vi "Command.vi"(7 "Cryo Idx":i32, 8 "error in (no error)":errorcluster, 9 "Options":string, 10 "Command":T1 items=["STATUS", "COOLER", "E", "ERROR", "KD", "KI", "KP", "LOGIN", "LOGOUT", "MODE", "P", "PWOUT", "SENSOR", "TC", "TEMP RJ", "TTARGET", "VERSION"], 11 "CryoCoolerAVC in":refnum<class "CryoCoolerAVC.lvclass">) -> (0 "error out":errorcluster, 2 "Response":string[](array[string]), 3 "CryoCoolerAVC out":refnum<class "CryoCoolerAVC.lvclass">)   [LabVIEW 2024, in "CryoCoolerAVC.lvclass"]
uses:
  CryoCoolerAVC.lvclass
  CryoCoolerAVC Command enum.ctl
  CryoCoolerAVC.lvclass/CryoCoolerAVC.ctl
  Cryo Cooler.lvclass
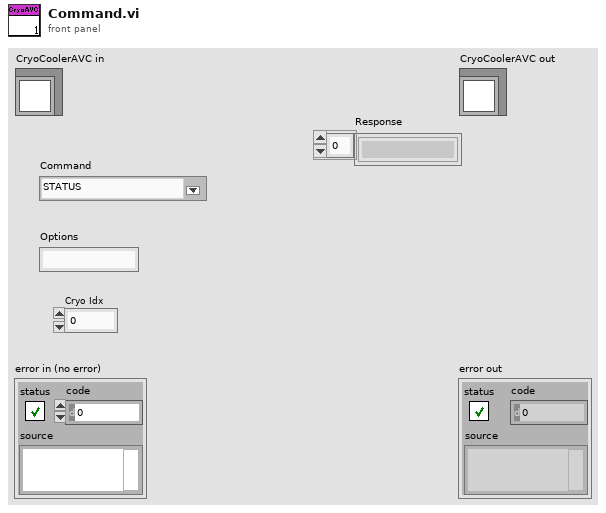
[diagram p1: front panel]
types:
  T1 = typedef "CryoCoolerAVC.lvclass/CryoCoolerAVC Command enum.ctl" = u16
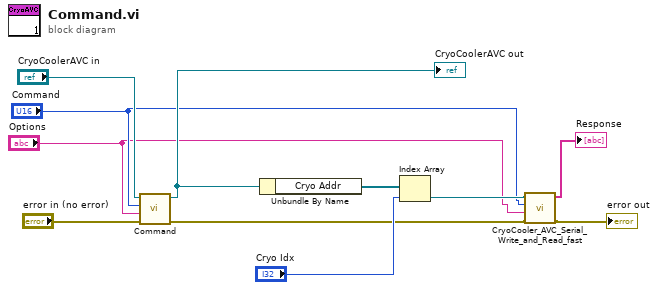
[diagram p0: block diagram]
diagram:
  n1 = call-parent "Command.vi"("error in (no error)"="error in (no error)", "Options"="Options", "Command"="Command", "Cryo Cooler in"="CryoCoolerAVC in") -> ("error out"=w7:errorcluster, "Cryo Cooler out"=w9:refnum<class "CryoCoolerAVC.lvclass">)  [unwired: 5 in, 1 out]
  "CryoCoolerAVC out" <- w9
  n2 = Unbundle By Name(w9) -> ("Cryo Addr"=w1:refnum<visa-resource-name>[])
  n3 = Index Array(array=w1, index="Cryo Idx") -> (element=w6:refnum<visa-resource-name>)
  n4 = call "CryoCooler_AVC_Serial_Write_and_Read_fast.vi"("error in (no error)"=w7, "Command Options"="Options", "Command"="Command", "VISA Resource (write)"=w6) -> ("error out"=→"error out":errorcluster, "read string array"=→"Response":string[])  [unwired: 5 in, 1 out]
